vi "Configure Analog Output.vi"(0 "VISA resource name":refnum<visa-resource-name>, 5 "Enable Analog Output (T: Enable)":bool=TRUE, 7 "Offset (0)":dbl, 9 "Gain (1)":dbl=1.0, 11 "error in (no error)":errorcluster, 12 "Enable Fixed Value Output (F: Disable)":bool, 13 "Fixed Value (0)":dbl) -> (4 "VISA resource name out":refnum<visa-resource-name>, 15 "error out":errorcluster)   [LabVIEW 2021, in "Agilent 34420.lvlib"]
doc: "Configures the settings for the Analog Out port at the back of the instrument.\n\nAnalog out port basically scales the readings taken at the measurement port and allows the user to keep track of or to graph the measurements. However a much better and easier way to do this would be taking the measurements using the <B>Read (Multiple Points)</B> or <B>Initiate</B> & <B>Fetch Multiple Points</B> VIs and then graphing the acquired data programmatically."
uses:
  <instrlib>/Agilent 34420/Agilent 34420.lvlib
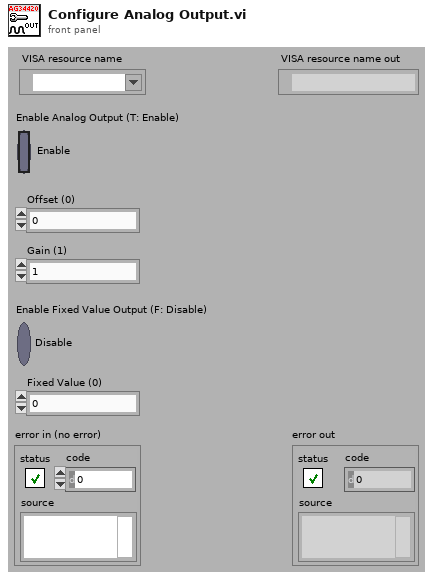
[diagram p1: front panel]
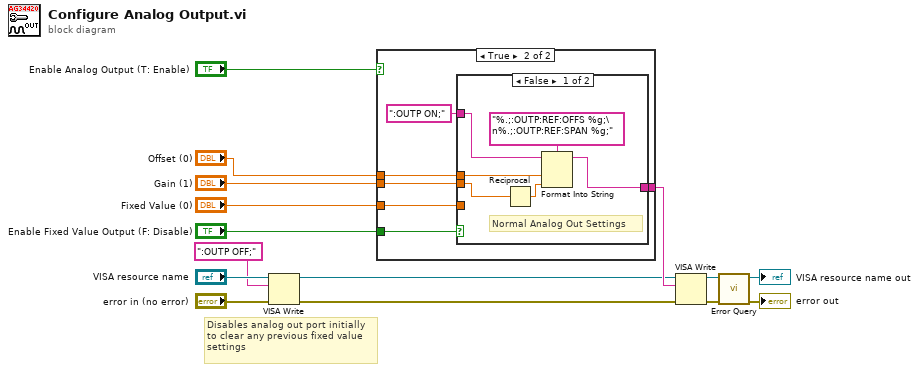
[diagram p0: block diagram]
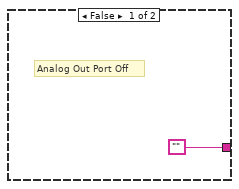
[diagram p2: hidden frame]
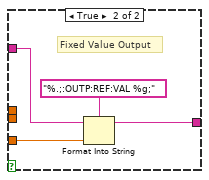
[diagram p3: hidden frame]
diagram:
  # "Disables analog out port initially\nto clear any previous fixed value\nsettings"
  n1 = VISA Write(VISA resource name="VISA resource name", write buffer=":OUTP OFF;", error in (no error)="error in (no error)") -> (VISA resource name out=w3:refnum<visa-resource-name>, error out=w2:errorcluster)  [unwired: 1 out]
  n2 = case shown="True" "Enable Analog Output (T: Enable)" {
    tunnel: "Enable Fixed Value Output (F: Disable)" -> [_ w22]
    tunnel: "Fixed Value (0)" -> [_ w20]
    tunnel: ["" w19] -> w8
    tunnel: "Offset (0)" -> [_ w18]
    tunnel: "Gain (1)" -> [_ w17]
    frame False {
      # "Analog Out Port Off"
    }
    frame True {
      n3 = case shown="False" w22 {
        tunnel: ":OUTP ON;" -> [w26 w32]
        tunnel: w20 -> [_ w31]
        tunnel: [w25 w29] -> w19
        tunnel: w18 -> [w27 _]
        tunnel: w17 -> [w24 _]
        frame False {
          # "Normal Analog Out Settings"
          n4 = Reciprocal(x=w24) -> (1/x=w23:dbl)
          n5 = Format Into String(format string="%.;:OUTP:REF:OFFS %g;\n%.;:OUTP:REF:SPAN %g;", initial string=w26, w27, w23) -> (resulting string=w25:string)  [unwired: 1 in, 1 out]
        }
        frame True {
          # "Fixed Value Output"
          n6 = Format Into String(format string="%.;:OUTP:REF:VAL %g;", initial string=w32, w31) -> (resulting string=w29:string)  [unwired: 1 in, 1 out]
        }
      }
    }
  }
  n7 = VISA Write(VISA resource name=w3, write buffer=w8, error in (no error)=w2) -> (VISA resource name out=w13:refnum<visa-resource-name>, error out=w12:errorcluster)  [unwired: 1 out]
  n8 = call <instrlib>:"Error Query.vi"("error in (no error)"=w12, "VISA resource name"=w13) -> ("error out"=→"error out":errorcluster, "VISA resource name out"=→"VISA resource name out":refnum<visa-resource-name>)  [unwired: 6 in, 2 out]
